vi "ChairTestAuto.vi"(0 "error in (no error)":errorcluster) -> ()   [LabVIEW 2014]
uses:
  <vilib>/Rock Robotics/WPI/RobotDrive/WPI_RobotDriveGetSetRefNum.vi
  <vilib>/Rock Robotics/WPI/RobotDrive/WPI_RobotDriveMecanumDrive_Cartesian.vi
  <vilib>/Rock Robotics/Network Tables/SD Write Numeric Array.vi
  <vilib>/Rock Robotics/Network Tables/SD Write String.vi
panel:
  out "error out":errorcluster
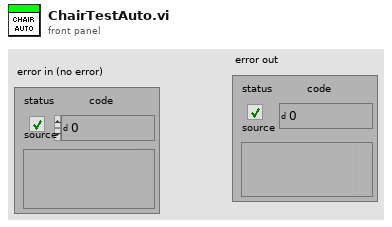
[diagram p1: front panel]
types:
  T1 = typedef "WPI_RobotDriveDevRef.ctl" = cluster{"DevStatus":errorcluster, "Motors[]":T2[], "Square Inputs":bool, "Max Output":dbl}
  T2 = typedef "WPI_MotorControlDeviceRef.ctl" = cluster{"DeviceStatus":errorcluster, "Type":T3, "PWM":cluster{"Controller":T4, "PWM Channel":T5, "DeadBand":T6}, "CAN":cluster{"Device Number":u8, "Control Mode":T7, "Semaphore":T8, "Max Vout":dbl, "TalonSRX Control Mode":T9}, "Invert":bool, "TransformRef":T10, "InvTransformRef":T10}
  T3 = typedef "WPI_MotorControlType.ctl" = enum16{"PWM", "CAN", "CANTalonSRX"}
  T4 = typedef "FPGA_TypedefDigitalModule.ctl" = enum16{"Controller 1"}
  T5 = typedef "FPGA_DIOPWMChannel.ctl" = enum8{"PWM 0", "PWM 1", "PWM 2", "PWM 3", "PWM 4", "PWM 5", "PWM 6", "PWM 7", "PWM 8", "PWM 9", "PWM MXP 0", "PWM MXP 1", "PWM MXP 2", "PWM MXP 3", "PWM MXP 4", "PWM MXP 5", "PWM MXP 6", "PWM MXP 7", "PWM MXP 8", "PWM MXP 9", "Invalid"}
  T6 = typedef "WPI_PWMDeadband.ctl" = cluster{"Name":string, "maxPositivePwm":i32, "minPositivePwm":i32, "centerPwm":i32, "maxNegativePwm":i32, "minNegativePwm":i32, "angularRange":u16}
  T7 = typedef "WPI_CANJaguar_ControlMode.ctl" = enum8{"Percent VBus", "Current", "Speed", "Position", "Voltage"}
  T8 = typedef "Semaphore RefNum" = refnum<k1>
  T9 = typedef "WPI_CANTalonSRX_APIControlMode.ctl" = enum8{"Percent VBus", "Speed", "Position", "Slave", "Unchanged / Invalid"}
  T10 = typedef "WPI_PWMTransform_ConPane.ctl" = refnum<vi>
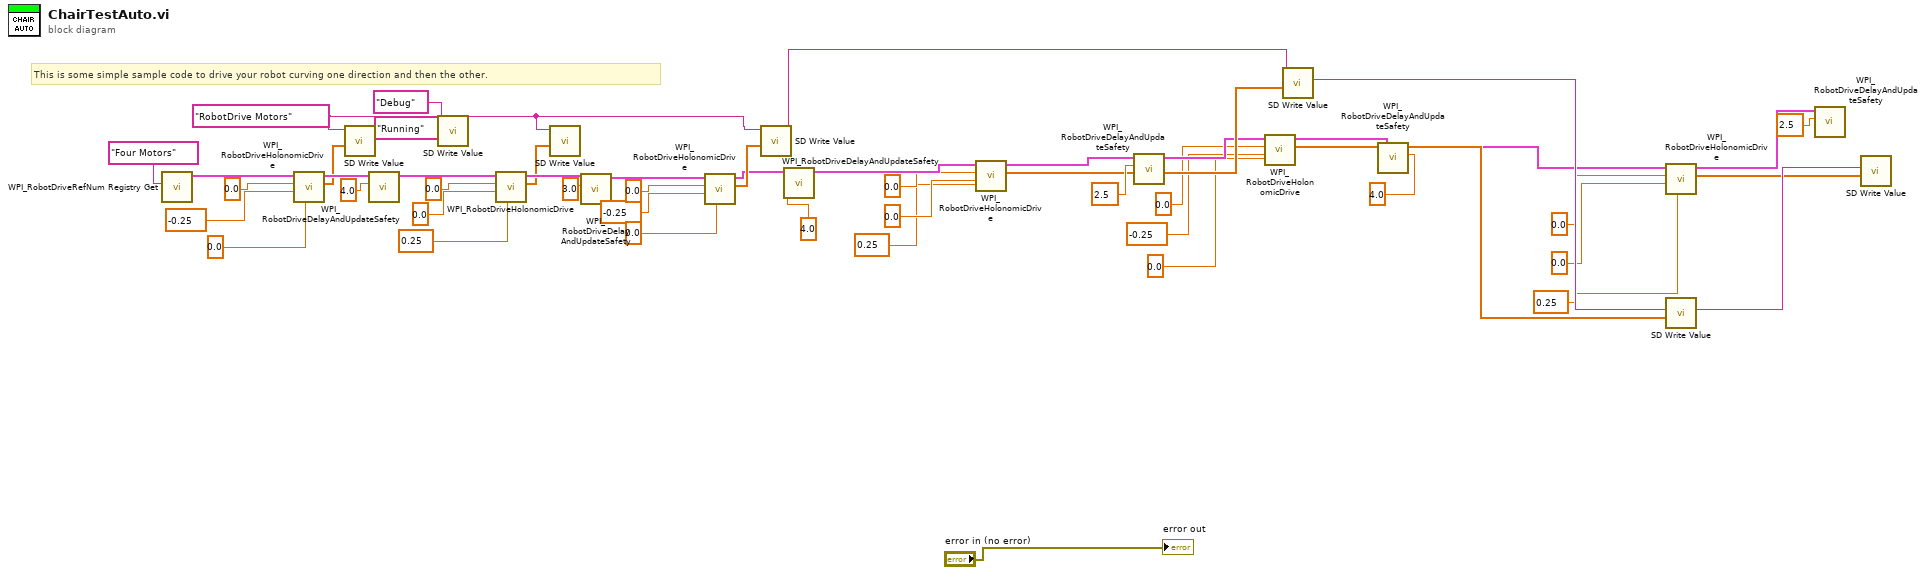
[diagram p0: block diagram]
diagram:
  w29 = "RobotDrive Motors" ("Name")
  # "This is some simple sample code to drive your robot curving one direction and then the other."
  n1 = call <vilib>:"WPI_RobotDriveRefNum Registry Get.vi"("refnum name"="Four Motors") -> ("RobotDriveDevRef"=w36:T1)  [unwired: 1 in, 9 out]
  n2 = call-poly <vilib>:"WPI_RobotDriveHolonomicDrive.vi"("Rotation"=0.0, "Y"=-0.25 ("X axis value"), "X"=0.0 ("X axis value"), "RobotDriveDevRef"=w36) -> ("Motor Values"=w32:dbl[], "RobotDriveDevRef"=w43:T1)  [unwired: 5 in, 1 out]
  n3 = call-poly <vilib>:"SD Write Value.vi"("Numeric Array"=w32, "Name"=w29) -> ()  [unwired: 8 in, 2 out]
  n4 = call <vilib>:"WPI_RobotDriveDelayAndUpdateSafety.vi"("Delay (s)"=4.0, "RobotDriveDevRef"=w43) -> ("RobotDriveDevRef 2"=w42:T1)  [unwired: 8 in, 1 out]
  n5 = call-poly <vilib>:"SD Write Value.vi"("String"="Running", "Name"="Debug") -> ()  [unwired: 8 in, 2 out]
  n6 = call-poly <vilib>:"WPI_RobotDriveHolonomicDrive.vi"("Rotation"=0.25, "Y"=0.0 ("X axis value"), "X"=0.0 ("X axis value"), "RobotDriveDevRef"=w42) -> ("Motor Values"=w31:dbl[], "RobotDriveDevRef"=w41:T1)  [unwired: 5 in, 1 out]
  n7 = call-poly <vilib>:"SD Write Value.vi"("Numeric Array"=w31, "Name"=w29) -> ()  [unwired: 8 in, 2 out]
  n8 = call <vilib>:"WPI_RobotDriveDelayAndUpdateSafety.vi"("Delay (s)"=3.0, "RobotDriveDevRef"=w41) -> ("RobotDriveDevRef 2"=w40:T1)  [unwired: 8 in, 1 out]
  n9 = call-poly <vilib>:"WPI_RobotDriveHolonomicDrive.vi"("Rotation"=0.0 ("X axis value"), "Y"=-0.25 ("X axis value"), "X"=0.0 ("X axis value"), "RobotDriveDevRef"=w40) -> ("Motor Values"=w30:dbl[], "RobotDriveDevRef"=w25:T1)  [unwired: 5 in, 1 out]
  n10 = call-poly <vilib>:"SD Write Value.vi"("Numeric Array"=w30, "Name"=w29) -> ("Table Prefix out"=w18:string)  [unwired: 8 in, 1 out]
  n11 = call <vilib>:"WPI_RobotDriveDelayAndUpdateSafety.vi"("Delay (s)"=4.0, "RobotDriveDevRef"=w25) -> ("RobotDriveDevRef 2"=w24:T1)  [unwired: 8 in, 1 out]
  n12 = call-poly <vilib>:"WPI_RobotDriveHolonomicDrive.vi"("Rotation"=0.25, "Y"=0.0, "X"=0.0, "RobotDriveDevRef"=w24) -> ("Motor Values"=w17:dbl[], "RobotDriveDevRef"=w20:T1)  [unwired: 5 in, 1 out]
  n13 = call <vilib>:"WPI_RobotDriveDelayAndUpdateSafety.vi"("Delay (s)"=2.5, "RobotDriveDevRef"=w20) -> ("RobotDriveDevRef 2"=w16:T1)  [unwired: 8 in, 1 out]
  n14 = call-poly <vilib>:"WPI_RobotDriveHolonomicDrive.vi"("Rotation"=0.0, "Y"=-0.25, "X"=0.0, "RobotDriveDevRef"=w16) -> ("Motor Values"=w10:dbl[], "RobotDriveDevRef"=w12:T1)  [unwired: 5 in, 1 out]
  n15 = call-poly <vilib>:"SD Write Value.vi"("Numeric Array"=w17, "Table Prefix"=w18) -> ("Table Prefix out"=w9:string)  [unwired: 8 in, 1 out]
  n16 = call <vilib>:"WPI_RobotDriveDelayAndUpdateSafety.vi"("Delay (s)"=4.0, "RobotDriveDevRef"=w12) -> ("RobotDriveDevRef 2"=w5:T1)  [unwired: 8 in, 1 out]
  n17 = call-poly <vilib>:"WPI_RobotDriveHolonomicDrive.vi"("Rotation"=0.25, "Y"=0.0, "X"=0.0, "RobotDriveDevRef"=w5) -> ("Motor Values"=w1:dbl[], "RobotDriveDevRef"=w4:T1)  [unwired: 5 in, 1 out]
  n18 = call-poly <vilib>:"SD Write Value.vi"("Numeric Array"=w10, "Table Prefix"=w9) -> ("Table Prefix out"=w2:string)  [unwired: 8 in, 1 out]
  n19 = call <vilib>:"WPI_RobotDriveDelayAndUpdateSafety.vi"("Delay (s)"=2.5, "RobotDriveDevRef"=w4) -> ()  [unwired: 8 in, 2 out]
  n20 = call-poly <vilib>:"SD Write Value.vi"("Numeric Array"=w1, "Table Prefix"=w2) -> ()  [unwired: 8 in, 2 out]
  "error out" <- "error in (no error)"
